vi "Process Messages.vi"(8 "error in (no error)":errorcluster, 10 "Channels in":refnum<data-value>[](array[refnum]), 11 "Message Queue":refnum<queue>) -> (0 "error out":errorcluster, 2 "Channels out":refnum<data-value>[](array[refnum]))   [LabVIEW 2020, in "G-Audio.lvlib" / "Mixer.lvclass"]
uses:
  Mixer.lvclass
  Controls/Message.ctl
  Controls/Command.ctl
  Channel/Channel.lvclass
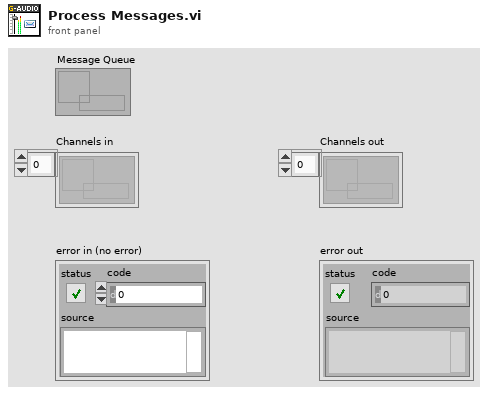
[diagram p1: front panel]
types:
  T1 = typedef "G-Audio.lvlib/Mixer.lvclass/Message.ctl" = cluster{"Command":T2, "Channel":i32, "Payload":variant}
  T2 = typedef "G-Audio.lvlib/Mixer.lvclass/Command.ctl" = enum16{"Channel Stop", "Channel Pause", "Channel Play", "Channel Volume", "Channel Unload"}
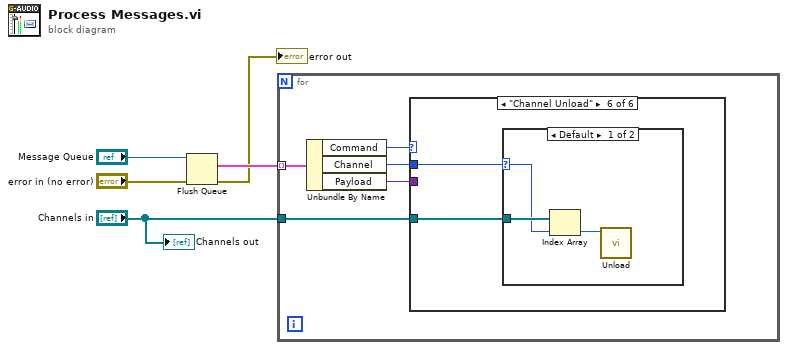
[diagram p0: block diagram]
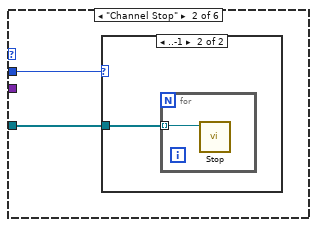
[diagram p3: hidden frame]
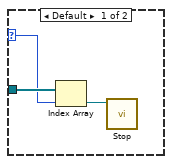
[diagram p4: hidden frame]
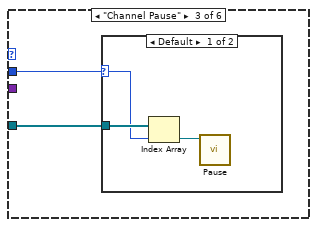
[diagram p5: hidden frame]
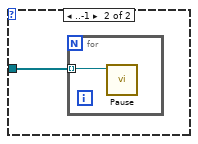
[diagram p6: hidden frame]
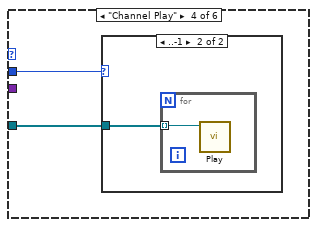
[diagram p7: hidden frame]
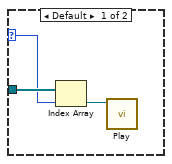
[diagram p8: hidden frame]
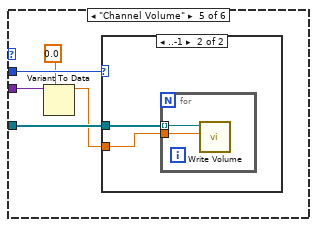
[diagram p9: hidden frame]
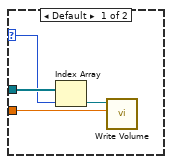
[diagram p10: hidden frame]
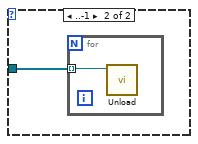
[diagram p11: hidden frame]
diagram:
  n1 = Flush Queue(queue="Message Queue", error in (no error)="error in (no error)") -> (remaining elements=w4:T1[], error out=→"error out":errorcluster)  [unwired: 1 out]
  n2 = for {
    tunnel: w4 -> [w10] mode=indexing
    tunnel: "Channels in" -> [w8]
    n3 = Unbundle By Name(w10) -> ("Command"=w9:T2, "Channel"=w7:i32, "Payload"=w6:variant)
    n4 = case shown="\"Channel Unload\"" w9 {
      tunnel: w8 -> [_ w12 w19 w26 w36 w46]
      tunnel: w7 -> [_ w11 w18 w25 w35 w45]
      tunnel: w6 -> [_ _ _ _ w34 _]
      frame Default {
      }
      frame "Channel Stop" {
        n5 = case shown="..-1" w11 {
          selector: w11 -> [w13 _]
          tunnel: w12 -> [w15 w16]
          frame Default {
            n6 = Index Array(array=w15, index=w13) -> (element=w14:refnum<data-value>)
            n7 = call "Stop.vi"("Channel in"=w14) -> ()  [unwired: 9 in, 2 out]
          }
          frame ..-1 {
            n8 = for {
              tunnel: w16 -> [w17] mode=indexing
              n9 = call "Stop.vi"("Channel in"=w17) -> ()  [unwired: 9 in, 2 out]
            }
          }
        }
      }
      frame "Channel Pause" {
        n10 = case shown="Default" w18 {
          selector: w18 -> [w20 _]
          tunnel: w19 -> [w22 w23]
          frame Default {
            n11 = Index Array(array=w22, index=w20) -> (element=w21:refnum<data-value>)
            n12 = call "Pause.vi"("Channel in"=w21) -> ()  [unwired: 9 in, 2 out]
          }
          frame ..-1 {
            n13 = for {
              tunnel: w23 -> [w24] mode=indexing
              n14 = call "Pause.vi"("Channel in"=w24) -> ()  [unwired: 9 in, 2 out]
            }
          }
        }
      }
      frame "Channel Play" {
        n15 = case shown="..-1" w25 {
          selector: w25 -> [w27 _]
          tunnel: w26 -> [w29 w30]
          frame Default {
            n16 = Index Array(array=w29, index=w27) -> (element=w28:refnum<data-value>)
            n17 = call "Play.vi"("Channel in"=w28) -> ()  [unwired: 9 in, 2 out]
          }
          frame ..-1 {
            n18 = for {
              tunnel: w30 -> [w31] mode=indexing
              n19 = call "Play.vi"("Channel in"=w31) -> ()  [unwired: 9 in, 2 out]
            }
          }
        }
      }
      frame "Channel Volume" {
        n20 = Variant To Data(type=0.0, Variant=w34) -> (data=w32:dbl)  [unwired: 1 in, 1 out]
        n21 = case shown="..-1" w35 {
          selector: w35 -> [w38 _]
          tunnel: w36 -> [w40 w42]
          tunnel: w32 -> [w37 w41]
          frame Default {
            n22 = Index Array(array=w40, index=w38) -> (element=w39:refnum<data-value>)
            n23 = call "Write Volume.vi"("Volume"=w37, "Channel in"=w39) -> ()  [unwired: 8 in, 2 out]
          }
          frame ..-1 {
            n24 = for {
              tunnel: w42 -> [w44] mode=indexing
              tunnel: w41 -> [w43]
              n25 = call "Write Volume.vi"("Volume"=w43, "Channel in"=w44) -> ()  [unwired: 8 in, 2 out]
            }
          }
        }
      }
      frame "Channel Unload" {
        n26 = case shown="Default" w45 {
          selector: w45 -> [w47 _]
          tunnel: w46 -> [w49 w50]
          frame Default {
            n27 = Index Array(array=w49, index=w47) -> (element=w48:refnum<data-value>)
            n28 = call "Unload.vi"("Channel in"=w48) -> ()  [unwired: 9 in, 2 out]
          }
          frame ..-1 {
            n29 = for {
              tunnel: w50 -> [w51] mode=indexing
              n30 = call "Unload.vi"("Channel in"=w51) -> ()  [unwired: 9 in, 2 out]
            }
          }
        }
      }
    }
  }
  "Channels out" <- "Channels in"
